vi "Abort.vi"(8 "error in (no error)":errorcluster, 11 "SMO":refnum<class "SMO.lvclass">) -> (0 "error out":errorcluster, 3 "SMO out":refnum<class "SMO.lvclass">)   [LabVIEW 2013, in "SMO.lvclass"]
doc: "---------------------------------------------------------------\nJKI State Machine Objects™\nhttp://jki.net/state-machine-objects/\nCopyright (C) 2005-2015, JKI <info@jki.net>\nALL RIGHTS RESERVED"
uses:
  SMO.lvclass
  SMO.lvclass/SMO.ctl
panel:
  # "For instructions on how to use the JKI State Machine Objects, examples and video tutorials, visit:\nhttp://jki.net/state-machine-objects/\n\nJKI State Machine Objects™\nhttp://jki.net/state-machine-objects/\nCopyright (C) 2005-2015, JKI <info@jki.net>\nALL RIGHTS RESERVED"
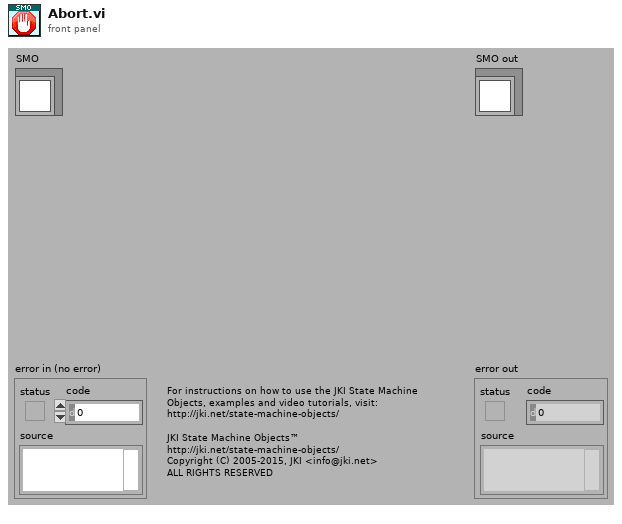
[diagram p1: front panel]
types:
  T1 = typedef "SMO.lvclass/PrivateData--Ref.ctl" = refnum<data-value>
  T2 = typedef "SMO.lvclass/PrivateData--Cluster.ctl" = cluster{"SMO Name":string, "Parent Call":T3, "Registered Processes":T4[], "Process Sync RendezVous":T5, "Process Error Notifier":refnum<notifier>, "Protected Events":T6, "Public Events":T7}
  T3 = typedef "SMO.lvclass/Parent Call--Enum.ctl" = enum16{"Allows parent to run", "Does not request parent to run"}
  T4 = typedef "SMO.lvclass/RegisteredProcessData--Cluster.ctl" = cluster{"Name":string, "Static VI Ref":refnum<vi>, "Running":bool}
  T5 = typedef "Rendezvous RefNum" = refnum<k1>
  T6 = typedef "SMO.lvclass/Protected Events.ctl" = cluster{"StopProcesses":refnum<user-event>, "AbortProcesses":refnum<user-event>}
  T7 = typedef "SMO.lvclass/Public Events.ctl" = cluster{"Error":refnum<user-event>}
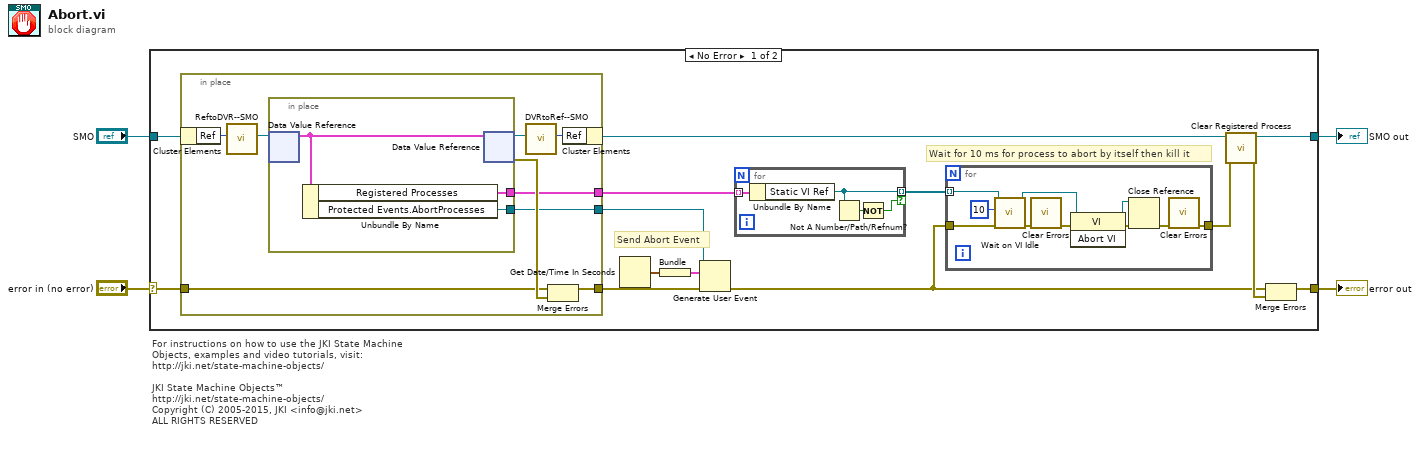
[diagram p0: block diagram]
diagram:
  # "For instructions on how to use the JKI State Machine Objects, examples and video tutorials, visit:\nhttp://jki.net/state-machine-objects/\n\nJKI State Machine Objects™\nhttp://jki.net/state-machine-objects/\nCopyright (C) 2005-2015, JKI <info@jki.net>\nALL RIGHTS RESERVED"
  n1 = case shown="No Error" "error in (no error)" {
    selector: "error in (no error)" -> [w17 w46]
    tunnel: [w12 w46] -> w3
    tunnel: [w10 w45] -> w1
    tunnel: "SMO" -> [w18 w45]
    frame No Error {
      # "Wait for 10 ms for process to abort by itself then kill it"
      # "Send Abort Event"
      n2 = in-place {
        in-place-border: w17 -> [w37]
        in-place-border: [w40] -> w13
        in-place-border: [w39] -> w14
        in-place-border: [w38] -> w7
        n3 = in-place-cluster #1(w18) -> ("Ref"=w36:u32)
        n4 = call "ReftoDVR--SMO.vi"("Ref"=w36) -> ("Ref"=w35:T1)  [unwired: 10 in]
        n5 = in-place {
          in-place-border: [w42] -> w39
          in-place-border: [w43] -> w38
          n6 = in-place-dvr #2(w35) -> (w44:T2)  [unwired: 1 out]
          n7 = Unbundle By Name(w44) -> ("Registered Processes"=w43:T4[], "Protected Events.AbortProcesses"=w42:refnum<user-event>)
          n8 = in-place-dvr #2(w44) -> (w34:T1, w41:errorcluster)
        }
        n9 = call "DVRtoRef--SMO.vi"("Ref"=w34) -> ("Ref"=w33:u32)  [unwired: 10 in]
        n10 = Merge Errors(w37, w41) -> (w40:errorcluster)
        n11 = in-place-cluster #1("Ref"=w33) -> (w11:refnum<class "SMO.lvclass">)
      }
      n12 = Get Date/Time In Seconds() -> (seconds since 1Jan1904=w15:timestamp)
      n13 = Bundle("seconds since 1Jan1904"=w15) -> (w16:cluster{"seconds since 1Jan1904":timestamp})  [unwired: 1 in]
      n14 = Generate User Event(user event=w14, event data cluster=w16, error in=w13) -> (error out=w5:errorcluster)  [unwired: 1 in, 1 out]
      n15 = for {
        tunnel: w7 -> [w20] mode=indexing
        tunnel: [w19] -> w6 mode=indexing if=w21
        n16 = Unbundle By Name(w20) -> ("Static VI Ref"=w19:refnum<vi>)
        n17 = Not A Number/Path/Refnum?(number/path/refnum=w19) -> (NaN/Path/Refnum?=w22:bool)
        n18 = Not(x=w22) -> (.not. x?=w21:bool)
      }
      n19 = for {
        tunnel: w5 -> [w32]
        tunnel: [w24] -> w8
        tunnel: w6 -> [w23] mode=indexing
        n20 = call "Wait on VI Idle.vi"("error in (no error)"=w32, "ms Timout (100ms)"=u32 10, "VI to Wait on"=w23) -> ("error out"=w30:errorcluster, "VI to Wait on dup"=w25:refnum<vi>)  [unwired: 6 in, 1 out]
        n21 = call <vilib>:"Clear Errors.vi"("error in (no error)"=w30) -> ("error out"=w29:errorcluster)  [unwired: 6 in]
        n22 = invoke class="VI" method="Abort VI"(reference=w25, error in=w29) -> (reference out=w26:refnum<vi>, error out=w28:errorcluster)  [unwired: 1 in, 1 out]
        n23 = Close Reference(reference=w26, error in (no error)=w28) -> (error out=w27:errorcluster)
        n24 = call <vilib>:"Clear Errors.vi"("error in (no error)"=w27) -> ("error out"=w24:errorcluster)  [unwired: 6 in]
      }
      n25 = call "Clear Registered Process.vi"("error in (no error)"=w8, "SMO"=w11) -> ("error out"=w9:errorcluster, "SMO out"=w10:refnum<class "SMO.lvclass">)  [unwired: 8 in]
      n26 = Merge Errors(w5, w9) -> (w12:errorcluster)
    }
    frame Error {
    }
  }
  "error out" <- w3
  "SMO out" <- w1
